vi "PDPLogging.vi"   [LabVIEW 2014]
uses:
  <vilib>/Utility/file.llb/Write To Spreadsheet File (string).vi
  <vilib>/Utility/file.llb/Write To Spreadsheet File (DBL).vi
types:
  T1 = cluster{"refnum name":string, "refnum name":string, "refnum name":string, "refnum name":string}
  T2 = typedef "WPI_AnalogChannelDevRef.ctl" = cluster{"DevStatus":errorcluster, "Controller":T3, "Analog Channel":T4}
  T3 = typedef "FPGA_TypedefAnalogModule.ctl" = enum16{"Controller 1"}
  T4 = typedef "FPGA_AIChannel.ctl" = enum8{"AI 0", "AI 1", "AI 2", "AI 3", "AI MXP 0", "AI MXP 1", "AI MXP 2", "AI MXP 3", "Invalid"}
  T5 = typedef "WPI_DriverStationRobotMode2.ctl" = enum16{"Autonomous Disabled", "Autonomous Enabled", "Teleop Disabled", "Teleop Enabled", "Disconnected", "Finish", "Test Disabled", "Test Enabled", "Emergency Stopped"}
  T6 = typedef "WPI_DriverStationPositionInfo.ctl" = enum16{"1", "2", "3"}
  T7 = typedef "WPI_DriverStationAllianceInfo.ctl" = enum16{"Red", "Blue", "Invalid"}
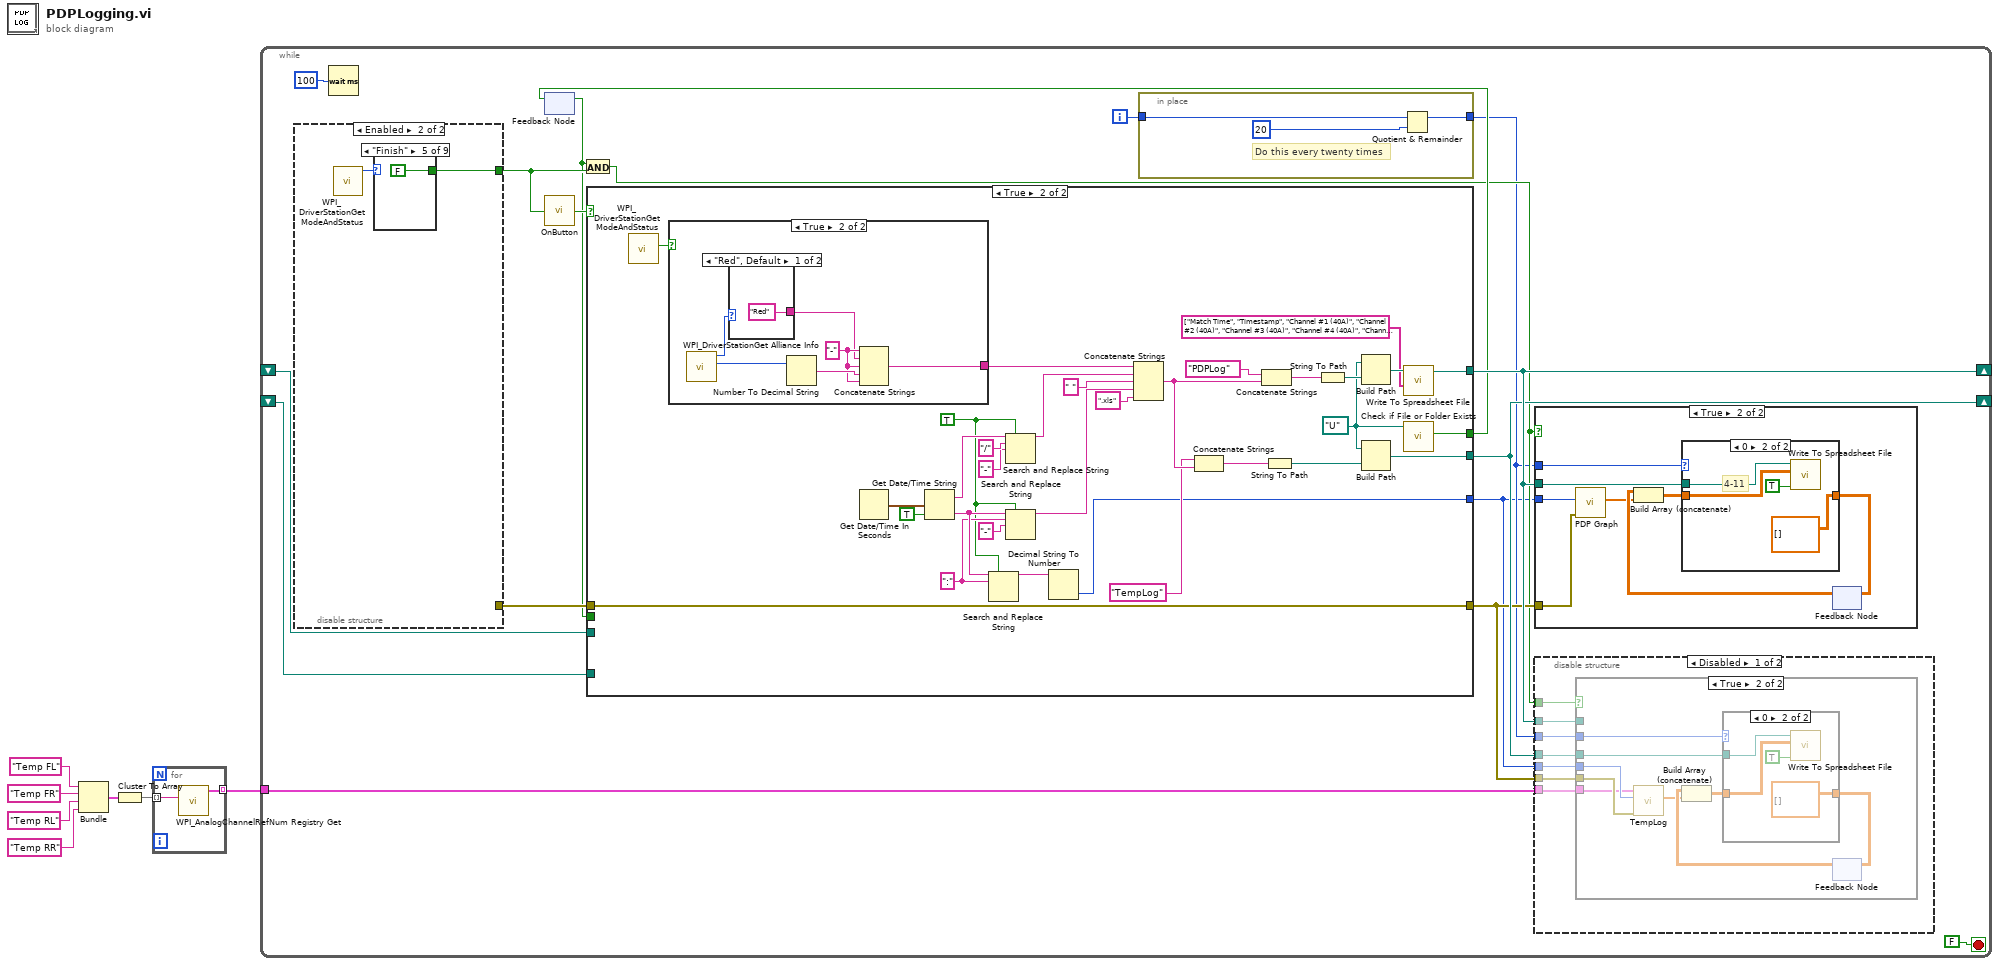
[diagram p0: block diagram]
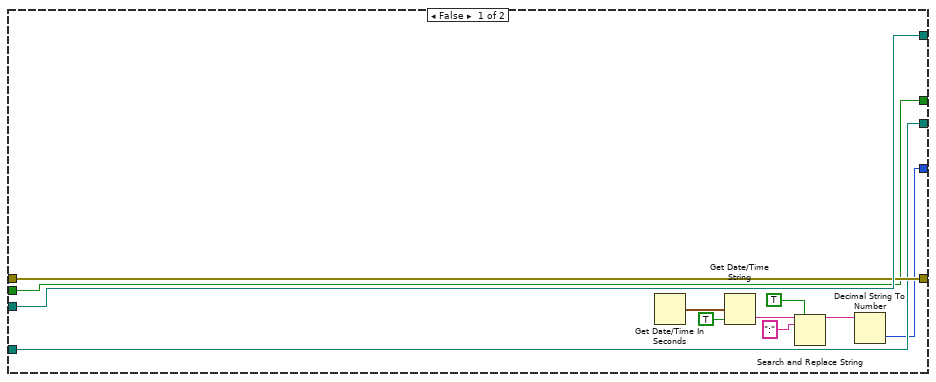
[diagram p5: hidden frame]
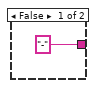
[diagram p6: hidden frame]
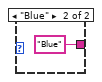
[diagram p7: hidden frame]
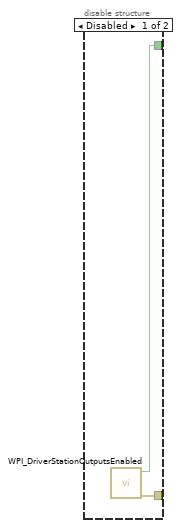
[diagram p10: hidden frame]
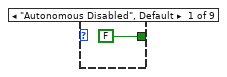
[diagram p11: hidden frame]
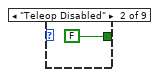
[diagram p12: hidden frame]
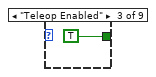
[diagram p13: hidden frame]
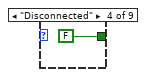
[diagram p14: hidden frame]
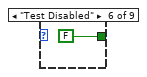
[diagram p15: hidden frame]
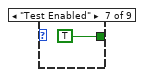
[diagram p16: hidden frame]
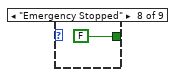
[diagram p17: hidden frame]
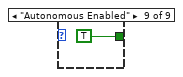
[diagram p18: hidden frame]
diagram:
  n1 = Bundle("refnum name"="Temp FL", "refnum name"="Temp FR", "refnum name"="Temp RL", "refnum name"="Temp RR") -> (w6:T1)  [unwired: 1 in]
  n2 = Cluster To Array(cluster=w6) -> (array=w7:string[])
  n3 = for {
    tunnel: w7 -> [w9] mode=indexing
    tunnel: [w8] -> w1 mode=indexing
    n4 = call <vilib>:"WPI_AnalogChannelRefNum Registry Get.vi"("refnum name"=w9) -> ("AIDeviceRef"=w8:T2)  [unwired: 9 in, 1 out]
  }
  n5 = while {
    shift-right: [w25] -> _
    shift-left: _ -> [w24]
    shift-right: [w21] -> _
    shift-left: _ -> [w20]
    tunnel: w1 -> [w10]
    i -> [w13]
    stop <- FALSE stop-if-true
    n6 = disable-structure shown="Enabled" {
      disable-tunnel: [w115 w117] -> w18
      disable-tunnel: [w116 _] -> w22
      frame Disabled {
        n7 = call <vilib>:"WPI_DriverStationOutputsEnabled.vi"() -> ("error out"=w116:errorcluster, "OutputsEnabled?"=w115:bool)  [unwired: 10 in]
      }
      frame Enabled {
        n8 = call <vilib>:"WPI_DriverStationGetModeAndStatus.vi"() -> ("Robot Mode"=w118:T5)  [unwired: 10 in, 1 out]
        n9 = case shown="\"Finish\"" w118 {
          tunnel: [FALSE FALSE TRUE FALSE FALSE FALSE TRUE FALSE TRUE] -> w117
          frame "Autonomous Disabled", Default {
          }
          frame "Teleop Disabled" {
          }
          frame "Teleop Enabled" {
          }
          frame "Disconnected" {
          }
          frame "Finish" {
          }
          frame "Test Disabled" {
          }
          frame "Test Enabled" {
          }
          frame "Emergency Stopped" {
          }
          frame "Autonomous Enabled" {
          }
        }
      }
    }
    n10 = Wait (ms)(milliseconds to wait=u32 100) -> ()  [unwired: 1 out]
    n11 = feedback #1() -> (w14:bool)  [unwired: 1 in]
    n12 = call "OnButton.vi"("Button"=w18) -> ("Value"=w26:bool)  [unwired: 1 in]
    n13 = And(x=w14, y=w18) -> (x .and. y?=w15:bool)
    n14 = case shown="True" w26 {
      tunnel: [w58 w60] -> w25
      tunnel: w24 -> [w58 _]
      tunnel: [w57 w66] -> w19
      tunnel: w22 -> [w57 w66]
      tunnel: [w56 w77] -> w21
      tunnel: w20 -> [w56 _]
      tunnel: [w55 w65] -> w16
      tunnel: w14 -> [w55 _]
      tunnel: [w54 w64] -> w11
      frame False {
        n15 = Get Date/Time In Seconds() -> (seconds since 1Jan1904=w50:timestamp)
        n16 = Get Date/Time String(seconds (now)=w50, want seconds? (F)=TRUE) -> (time string=w52:string)  [unwired: 1 in, 1 out]
        n17 = Search and Replace String(replace all?=TRUE ("replace all? (F)"), input string=w52, search string=":") -> (result string=w53:string)  [unwired: 5 in, 3 out]
        n18 = Decimal String To Number(string=w53) -> (number=w54:i32)  [unwired: 2 in, 1 out]
      }
      frame True {
        w71 = ":" ("search string")
        w70 = TRUE ("replace all? (F)")
        w79 = path "U:/" ("base path")
        n19 = call <vilib>:"WPI_DriverStationGetModeAndStatus.vi"() -> ("FMS Attached"=w89:bool)  [unwired: 10 in, 1 out]
        n20 = case shown="True" w89 {
          tunnel: ["-" ("string") w93] -> w88
          frame False {
          }
          frame True {
            w94 = "-" ("string")
            n21 = call <vilib>:"WPI_DriverStationGet Alliance Info.vi"() -> ("Position"=w96:T6, "Alliance"=w91:T7)  [unwired: 10 in]
            n22 = case shown="\"Red\", Default" w91 {
              tunnel: ["Red" "Blue"] -> w92
              frame "Red", Default {
              }
              frame "Blue" {
              }
            }
            n23 = Number To Decimal String(number=w96) -> (decimal integer string=w95:string)  [unwired: 1 in]
            n24 = Concatenate Strings(w94, w92, w94, w95, w94) -> (w93:string)
          }
        }
        n25 = Get Date/Time In Seconds() -> (seconds since 1Jan1904=w86:timestamp)
        n26 = Get Date/Time String(seconds (now)=w86, want seconds? (F)=TRUE) -> (date string=w76:string, time string=w72:string)  [unwired: 1 in]
        n27 = Search and Replace String(replace all?=w70, input string=w72, search string=w71) -> (result string=w63:string)  [unwired: 5 in, 3 out]
        n28 = Search and Replace String(replace all?=w70, input string=w76, search string="/", replace string="-" ("replace string (\"\")")) -> (result string=w73:string)  [unwired: 4 in, 3 out]
        n29 = Search and Replace String(replace all?=w70, input string=w72, search string=w71, replace string="-") -> (result string=w69:string)  [unwired: 4 in, 3 out]
        n30 = Decimal String To Number(string=w63) -> (number=w64:i32)  [unwired: 2 in, 1 out]
        n31 = Concatenate Strings(w88, w73, " " ("string"), w69, ".xls" ("string")) -> (w82:string)
        n32 = Concatenate Strings("TempLog" ("string"), w82) -> (w81:string)
        n33 = Concatenate Strings("PDPLog", w82) -> (w84:string)
        n34 = String To Path(string=w81) -> (path=w80:path)
        n35 = String To Path(string=w84) -> (path=w87:path)
        n36 = Build Path(base path=w79, name or relative path=w87) -> (appended path=w61:path)
        n37 = Build Path(base path=w79, name or relative path=w80) -> (appended path=w77:path)
        n38 = call-poly <vilib>:"Write To Spreadsheet File.vi"("1D data"=string[] ["Match Time", "Timestamp", "Channel #1 (40A)", "Channel #2 (40A)", "Channel #3 (40A)", "Channel #4 (40A)", "Channel #13 (40A)", "Channel #14 (40A)", "Channel #15 (40A)", "Channel #16 (40A)", "Channel #5 (20/30A)", "Channel #6 (20/30A)", "Channel #7 (20/30A)", "Channel #8 (20/30A)", "Channel #9 (20/30A)", "Channel #10 (20/30A)", "Channel #11 (20/30A)", "Channel #12 (20/30A)", "PDP Voltage"] ("appended array"), "file path (dialog if empty)"=w61) -> ("new file path (Not A Path if cancelled)"=w60:path)  [unwired: 6 in]
        n39 = call <vilib>:"Check if File or Folder Exists.vi"("path"=w79) -> ("file or folder exists?"=w65:bool)  [unwired: 8 in, 2 out]
      }
    }
    n40 = feedback-in #1(w16) -> ()
    n41 = in-place {
      in-place-border: w13 -> [w101]
      in-place-border: [w100] -> w12
      # "Do this every twenty times"
      n42 = Quotient & Remainder(x=w101, y=20) -> (x-y*floor(x/y)=w100:i32)  [unwired: 1 out]
    }
    n43 = case shown="True" w15 {
      tunnel: w19 -> [_ w109]
      tunnel: w25 -> [_ w108]
      tunnel: w11 -> [_ w106]
      tunnel: w12 -> [_ w105]
      frame False {
      }
      frame True {
        n44 = call "PDP Graph.vi"("error in"=w109, "Timestamp"=w106) -> ("Current"=w102:dbl[])  [unwired: 8 in, 1 out]
        n45 = feedback #2() -> (w103:dbl[][])  [unwired: 1 in]
        n46 = Build Array (concatenate)(w103, w102) -> (w104:dbl[][])
        n47 = case shown="0" w105 {
          tunnel: w108 -> [_ w114]
          tunnel: w104 -> [w110 w112]
          tunnel: [w110 dbl[][] []] -> w107
          frame 1, Default {
          }
          frame 0 {
            # "4-11"
            n48 = call-poly <vilib>:"Write To Spreadsheet File.vi"("append to file? (new file:F)"=TRUE, "2D data"=w112, "file path (dialog if empty)"=w114) -> ()  [unwired: 5 in, 1 out]
          }
        }
        n49 = feedback-in #2(w107) -> ()
      }
    }
    n50 = disable-structure shown="Disabled" {
      disable-tunnel: w25 -> [w33 _]
      disable-tunnel: w21 -> [w32 _]
      disable-tunnel: w19 -> [w31 _]
      disable-tunnel: w15 -> [w30 _]
      disable-tunnel: w12 -> [w29 _]
      disable-tunnel: w11 -> [w28 _]
      disable-tunnel: w10 -> [w27 _]
      frame Disabled {
        n51 = case shown="True" w30 {
          tunnel: w31 -> [_ w39]
          tunnel: w32 -> [_ w37]
          tunnel: w33 -> [_ _]
          tunnel: w29 -> [_ w42]
          tunnel: w28 -> [_ w41]
          tunnel: w27 -> [_ w38]
          frame False {
          }
          frame True {
            n52 = call "TempLog.vi"("error in (no error)"=w39, "Timestamp"=w41, "Temp Refs"=w38) -> ("Temp"=w34:dbl[])  [unwired: 7 in, 1 out]
            n53 = feedback #3() -> (w35:dbl[][])  [unwired: 1 in]
            n54 = Build Array (concatenate)(w35, w34) -> (w36:dbl[][])
            n55 = case shown="0" w42 {
              tunnel: w37 -> [_ w47]
              tunnel: w36 -> [w43 w45]
              tunnel: [w43 dbl[][] []] -> w40
              frame 1, Default {
              }
              frame 0 {
                n56 = call-poly <vilib>:"Write To Spreadsheet File.vi"("append to file? (new file:F)"=TRUE, "2D data"=w45, "file path (dialog if empty)"=w47) -> ()  [unwired: 5 in, 1 out]
              }
            }
            n57 = feedback-in #3(w40) -> ()
          }
        }
      }
      frame Enabled {
      }
    }
  }
